vi "Harmonic Peak finder.vi"(2 "end position":i32(slide)=10 scale=0.0..20.0, 3 "start position":i32(slide)=5 scale=0.0..10.0, 4 "width":i32(slide)=4 scale=0.0..4.0, 5 "Input":dbl[][](array[numeric])) -> (0 "first harmonic index":i32, 1 "Peaks":dbl[](array[numeric]))   [LabVIEW 2009]
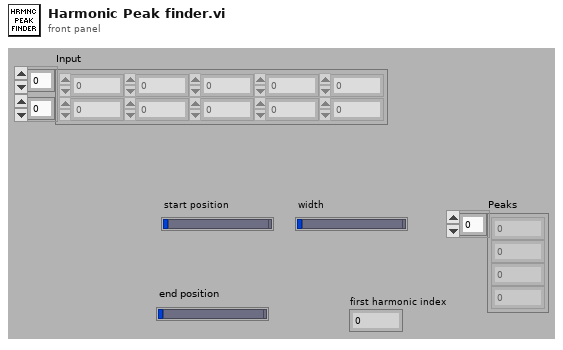
[diagram p1: front panel]
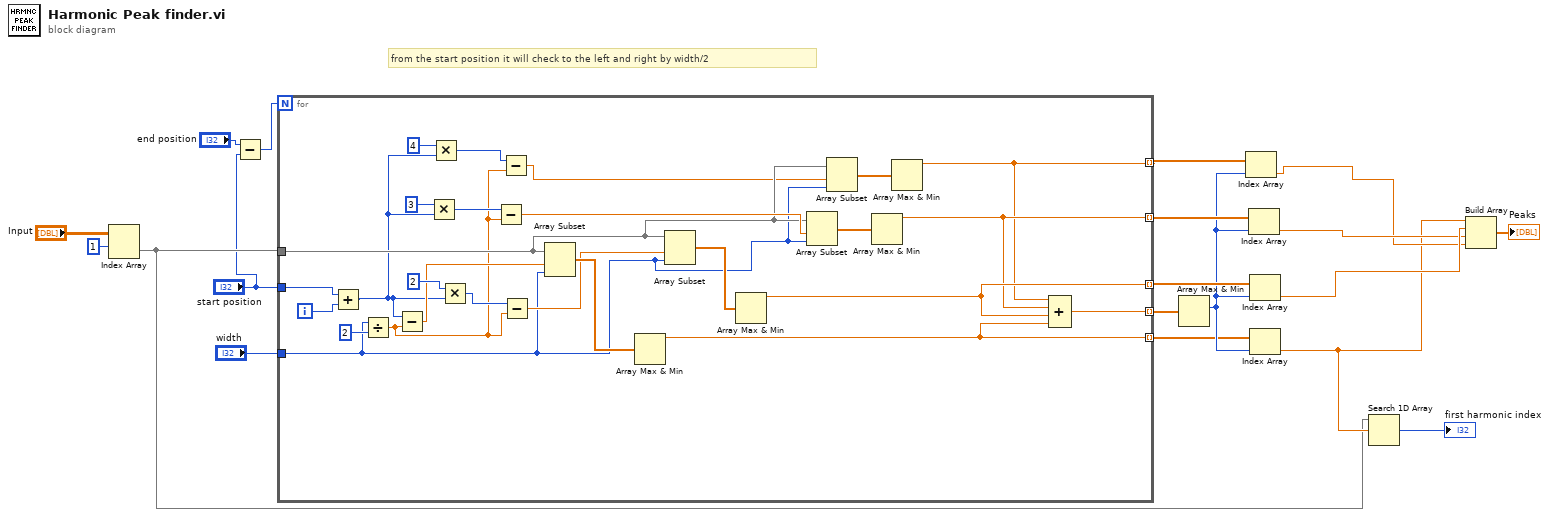
[diagram p0: block diagram]
diagram:
  # "from the start position it will check to the left and right by width/2"
  n1 = Index Array(array="Input", index (row)=1) -> (element=w4:dbl[])  [unwired: 1 in]
  n2 = Subtract(x="end position", y="start position") -> (x-y=w1:i32)
  n3 = for {
    N: w1 -> [_]
    tunnel: "width" -> [w26]
    tunnel: w4 -> [w27]
    tunnel: "start position" -> [w37]
    tunnel: [w36] -> w17 mode=indexing
    tunnel: [w35] -> w6 mode=indexing
    tunnel: [w34] -> w16 mode=indexing
    tunnel: [w29] -> w18 mode=indexing
    tunnel: [w20] -> w19 mode=indexing
    i -> [w38]
    n4 = Add(x=w37, y=w38) -> (x+y=w25:i32)
    n5 = Divide(x=w26, y=2) -> (x/y=w23:dbl)
    n6 = Subtract(x=w25, y=w23) -> (x-y=w42:dbl)
    n7 = Multiply(x=3, y=w25) -> (x*y=w32:i32)
    n8 = Multiply(x=4, y=w25) -> (x*y=w22:i32)
    n9 = Multiply(x=2, y=w25) -> (x*y=w41:i32)
    n10 = Subtract(x=w32, y=w23) -> (x-y=w31:dbl)
    n11 = Subtract(x=w22, y=w23) -> (x-y=w21:dbl)
    n12 = Subtract(x=w41, y=w23) -> (x-y=w40:dbl)
    n13 = Array Subset(array=w27, index=w42, length=w26) -> (w43:dbl[])
    n14 = Array Max & Min(array=w43) -> (max value=w35:dbl)  [unwired: 3 out]
    n15 = Array Subset(array=w27, index=w40, length=w26) -> (w44:dbl[])
    n16 = Array Max & Min(array=w44) -> (max value=w36:dbl)  [unwired: 3 out]
    n17 = Array Subset(array=w27, index=w31, length=w26) -> (w30:dbl[])
    n18 = Array Subset(array=w27, index=w21, length=w26) -> (w28:dbl[])
    n19 = Array Max & Min(array=w30) -> (max value=w29:dbl)  [unwired: 3 out]
    n20 = Array Max & Min(array=w28) -> (max value=w20:dbl)  [unwired: 3 out]
    n21 = Compound Arithmetic op=ADD(w20, w29, w36, w35) -> (w34:dbl)
  }
  n22 = Array Max & Min(array=w16) -> (max index (indices)=w14:i32)  [unwired: 3 out]
  n23 = Index Array(array=w19, index=w14) -> (element=w10:dbl)
  n24 = Index Array(array=w18, index=w14) -> (element=w11:dbl)
  n25 = Index Array(array=w17, index=w14) -> (element=w12:dbl)
  n26 = Index Array(array=w6, index=w14) -> (element=w5:dbl)
  n27 = Search 1D Array(1D array=w4, element=w5) -> (index of element=→"first harmonic index":i32)  [unwired: 1 in]
  n28 = Build Array(w5, w12, w11, w10) -> (→"Peaks":dbl[])
